vi "EX 8-1 LCD Hello World 4-bit.vi"() -> ()   [LabVIEW 2011, in "LabVIEW Interface for Arduino.lvlib"]
doc: "Writes the text on the front panel to the LCD Screen using 4-bit mode."
uses:
  <vilib>/LabVIEW Interface for Arduino/LabVIEW Interface for Arduino.lvlib
  <vilib>/LabVIEW Interface for Arduino/Type Defs/LCD Pin Config 4 bit.ctl
panel:
  in  "Rows":u8=2
  in  "Columns":u8=16
  in  "LCD Text":string="Hello World"
  in  "LCD Pin Config 4 Bit":T1={"RS"=12, "RW"=255, "Enable"=11, "D4"=5, "D5"=4, "D6"=3, "D7"=2, "LCD"=10}
  # "Configuration"
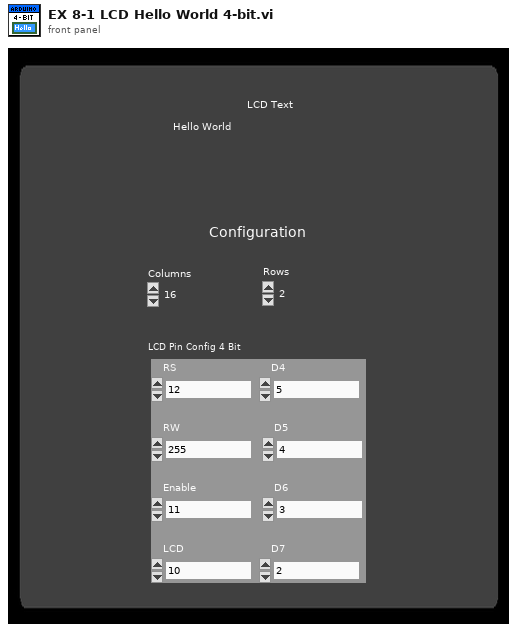
[diagram p1: front panel]
types:
  T1 = typedef "LabVIEW Interface for Arduino.lvlib/LCD Pin Config 4 bit.ctl" = cluster{"RS":u8, "RW":u8, "Enable":u8, "D4":u8, "D5":u8, "D6":u8, "D7":u8, "LCD":u8}
  T2 = enum8{"String", "Binary", "Decimal", "Octal", "Hexadecimal"}
  T3 = typedef "LabVIEW Interface for Arduino.lvlib/Arduino Resource.ctl" = cluster{"VISA resource":refnum<visa-resource-name>, "Board Type":T4, "Connection Type":enum8{"USB / Serial"}, "Bytes Per Packet (15)":u8}
  T4 = typedef "LabVIEW Interface for Arduino.lvlib/Board Type.ctl" = enum16{"Uno", "Dimuelanove w/Atmega 328", "Mega 2560"}
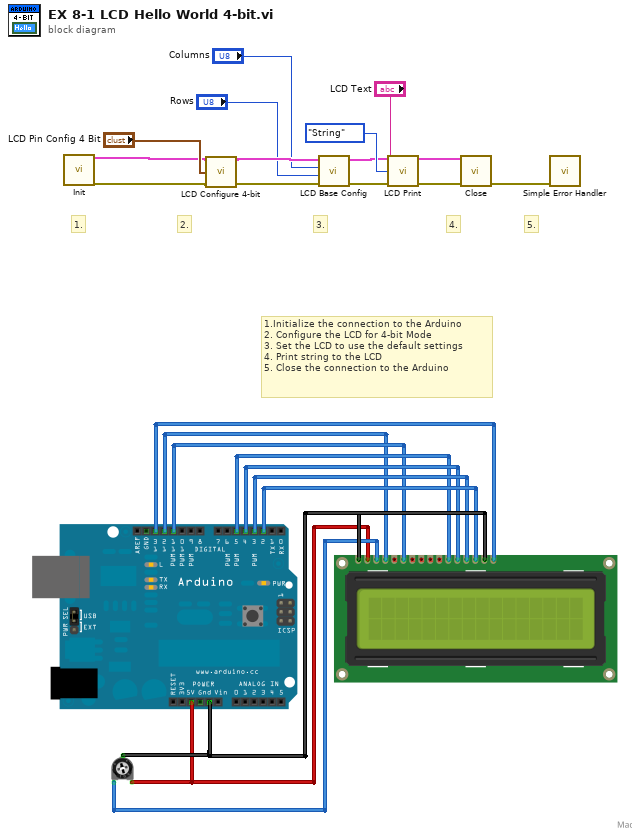
[diagram p0: block diagram]
diagram:
  # "1.Initialize the connection to the Arduino\n2. Configure the LCD for 4-bit Mode\n3. Set the LCD to use the default settings\n4. Print string to the LCD\n5. Close the connection to the Arduino"
  # "5."
  # "4."
  # "3."
  # "2."
  # "1."
  n1 = call <vilib>:"Init.vi"() -> ("Arduino Resource"=w5:T3, "error out"=w7:errorcluster)  [unwired: 18 in]
  n2 = call <vilib>:"LCD Configure 4-bit.vi"("Arduino Resource"=w5, "LCD Pin Config 4 Bit"="LCD Pin Config 4 Bit", "error in"=w7) -> ("Arduino Resource"=w4:T3, "error out"=w8:errorcluster)  [unwired: 11 in]
  n3 = call <vilib>:"LCD Base Config.vi"("error in (no error)"=w8, "Rows"="Rows", "Columns"="Columns", "Arduino Resource in"=w4) -> ("error out"=w9:errorcluster, "Arduino Resource out"=w10:T3)  [unwired: 6 in]
  n4 = call <vilib>:"LCD Print.vi"("Arduino Resource"=w10, "Data"="LCD Text", "Base (String)"=T2."String", "error out"=w9) -> ("Arduino Resource"=w13:T3, "error out"=w12:errorcluster)  [unwired: 10 in]
  n5 = call <vilib>:"Close.vi"("Arduino Resource"=w13, "error in"=w12) -> ("error out"=w11:errorcluster)  [unwired: 13 in]
  n6 = call <vilib>:"Simple Error Handler.vi"("error in (no error)"=w11) -> ()  [unwired: 4 in, 5 out]
